vi "Ctor.vi"(8 "error in (no error)":errorcluster, 11 "Item Summary in":refnum<class "Item Summary.lvclass">) -> (0 "error out":errorcluster, 3 "Item Summary out":refnum<class "Item Summary.lvclass">)   [LabVIEW 2020, in "Item Summary.lvclass"]
uses:
  Item Summary.lvclass
  Item/Ingredient.ctl
  Item/Item.lvclass
  Item Summary.lvclass/Item Summary.ctl
  <vilib>/IlluminatedG/IG OOPanel/OOPanel/ArrayPanel/ArrayPanel.lvclass
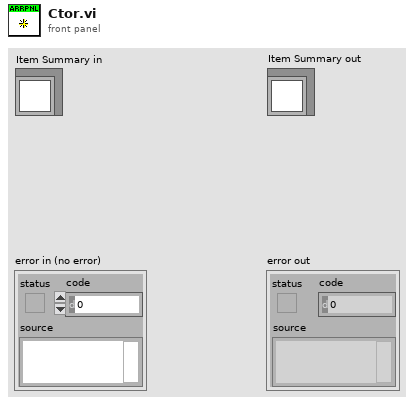
[diagram p1: front panel]
types:
  T1 = typedef "Item.lvclass/Ingredient.ctl" = cluster{"Item":refnum<class "Item.lvclass">, "Qty":dbl}
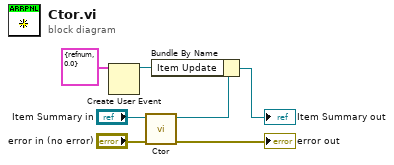
[diagram p0: block diagram]
diagram:
  n1 = Create User Event(user event datatype=T1 {"Item"=refnum, "Qty"=0.0} ("Ingredient")) -> (user event=w1:refnum<user-event>)  [unwired: 1 in, 1 out]
  n2 = call-parent "Ctor.vi"("error in (no error)"="error in (no error)", "ArrayPanel in"="Item Summary in") -> ("error out"=→"error out":errorcluster, "ArrayPanel out"=w3:refnum<class "Item Summary.lvclass">)  [unwired: 8 in]
  n3 = Bundle By Name(cluster=w3, "Item Update"=w1) -> (→"Item Summary out":refnum<class "Item Summary.lvclass">)
